vi "Config PM Modulation.vi"(0 "VISA Resource Name":refnum<visa-resource-name>, 1 "Path (0:1)":enum16{"1", "2"}(ring), 2 "Status (T:ON)":bool=TRUE, 3 "EXT Source Coupling (T:AC)":bool=TRUE, 4 "PM Deviation Couple (F:OFF)":bool, 5 "error in (no error)":errorcluster {"code" format="%.0x"}, 6 "PM Deviation (0.0)":dbl format="%.3f", 7 "Dual/Swept Parameters":T1={"Alt Frequency (400.0)"=400.0, "Alt Freq Amplitude (50.0)"=50.0, "Sweep Time (100.0)"=100.0, "Sweep Trigger (0:IMMEDIATE)"=enum."IMMEDIATE"} {"Sweep Time (100.0)" format="%.1f"; "Alt Freq Amplitude (50.0)" format="%.1f"; "Alt Frequency (400.0)" format="%.1f"}, 8 "PM Source (0:Internal)":enum16{"INTERNAL", "EXT1", "EXT2"}(ring), 9 "Bandwidth (T:NORMAL)":bool=TRUE, 10 "PM Rate (400.0)":dbl=400.0 format="%.1f", 12 "PM Waveform (0:SINE)":T2(ring)) -> (14 "VISA Resource Name Out":refnum<visa-resource-name>, 19 "error out":errorcluster {"code" format="%.0x"})   [LabVIEW 2012, in "Agilent ESG Series.lvlib"]
doc: "This VI is used to set the modulation controls and the parameters associated with phase modulated signals."
uses:
  <instrlib>/Agilent ESG Series/Agilent ESG Series.lvlib
panel:
  # "NORMAL"
  # "HIGH"
  # "ON"
  # "OFF"
  # "AC"
  # "DC"
  # "ON"
  # "OFF"
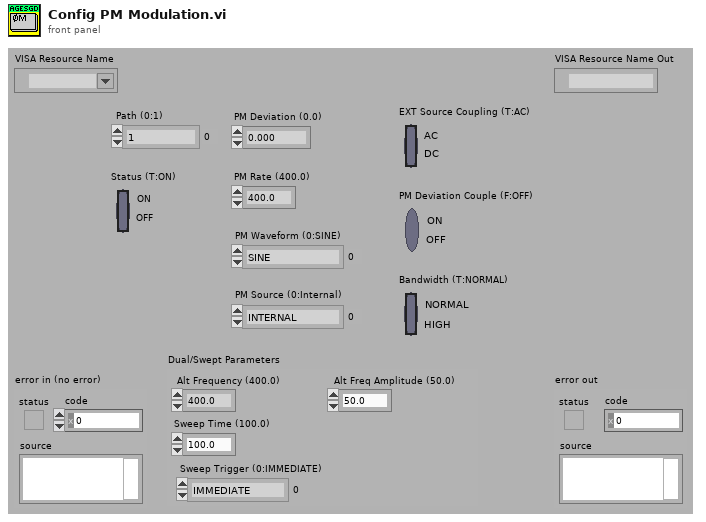
[diagram p1: front panel]
types:
  T1 = cluster{"Alt Frequency (400.0)":dbl, "Alt Freq Amplitude (50.0)":dbl, "Sweep Time (100.0)":dbl, "Sweep Trigger (0:IMMEDIATE)":enum16{"IMMEDIATE", "BUS", "EXTERNAL", "KEY"}}
  T2 = enum16{"SINE", "TRIANGLE", "SQUARE", "RAMP", "NOISE", "DUAL SINE", "SWEPT SINE"}
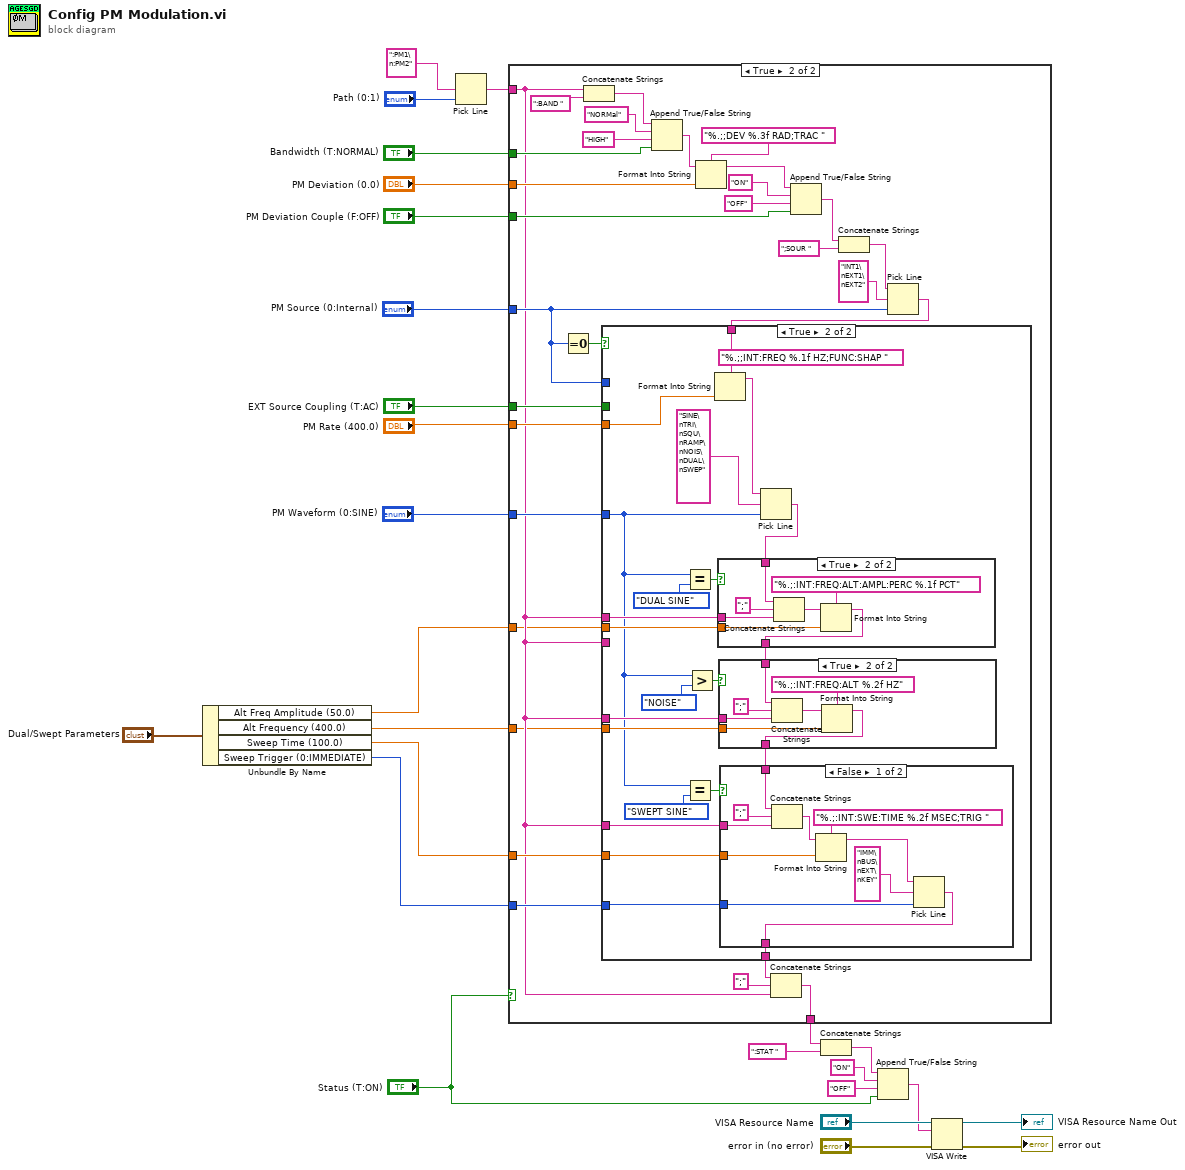
[diagram p0: block diagram]
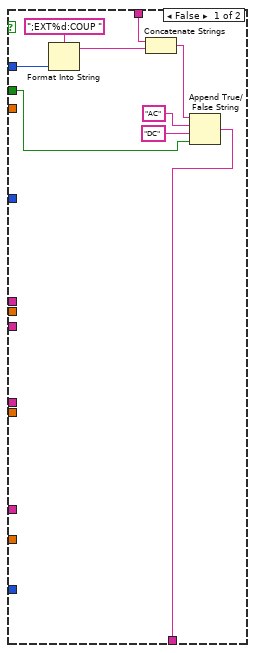
[diagram p3: hidden frame]
diagram:
  n1 = Unbundle By Name("Dual/Swept Parameters") -> ("Alt Freq Amplitude (50.0)"=w3:dbl, "Alt Frequency (400.0)"=w4:dbl, "Sweep Time (100.0)"=w1:dbl, "Sweep Trigger (0:IMMEDIATE)"=w2:enum16{"IMMEDIATE", "BUS", "EXTERNAL", "KEY"})
  n2 = Pick Line(multi-line string=":PM1\n:PM2" ("true string"), line index="Path (0:1)") -> (output string=w9:string)  [unwired: 1 in]
  n3 = case shown="True" "Status (T:ON)" {
    tunnel: "Bandwidth (T:NORMAL)" -> [_ w57]
    tunnel: w9 -> [w27 w30]
    tunnel: [w27 w40] -> w14
    tunnel: w1 -> [_ w38]
    tunnel: w2 -> [_ w37]
    tunnel: "PM Waveform (0:SINE)" -> [_ w36]
    tunnel: "PM Rate (400.0)" -> [_ w35]
    tunnel: "EXT Source Coupling (T:AC)" -> [_ w34]
    tunnel: "PM Source (0:Internal)" -> [_ w33]
    tunnel: "PM Deviation Couple (F:OFF)" -> [_ w32]
    tunnel: "PM Deviation (0.0)" -> [_ w31]
    tunnel: w3 -> [_ w29]
    tunnel: w4 -> [_ w28]
    frame False {
    }
    frame True {
      n4 = Equal To 0?(x=w33) -> (x = 0?=w43:bool)
      n5 = Concatenate Strings(w30, ":BAND ") -> (w55:string)
      n6 = Append True/False String(1:w57, 2:"HIGH" ("false string"), 3:"NORMal" ("true string"), 4:w55) -> (0:w56:string)
      n7 = Format Into String(format string="%.;;DEV %.3f RAD;TRAC ", initial string=w56, w31) -> (resulting string=w48:string)  [unwired: 1 in, 1 out]
      n8 = Append True/False String(1:w32, 2:"OFF" ("false string"), 3:"ON" ("true string"), 4:w48) -> (0:w47:string)
      n9 = Concatenate Strings(w47, ";SOUR ") -> (w45:string)
      n10 = Pick Line(string ("")=w45, multi-line string="INT1\nEXT1\nEXT2", line index=w33) -> (output string=w42:string)
      n11 = case shown="True" w43 {
        tunnel: w42 -> [w65 w89]
        tunnel: [w62 w82] -> w39
        tunnel: w33 -> [w61 _]
        tunnel: w34 -> [w58 _]
        tunnel: w35 -> [_ w88]
        tunnel: w36 -> [_ w69]
        tunnel: w37 -> [_ w80]
        tunnel: w38 -> [_ w81]
        tunnel: w30 -> [_ _]
        tunnel: w30 -> [_ w79]
        tunnel: w30 -> [_ w73]
        tunnel: w30 -> [_ w72]
        tunnel: w29 -> [_ w71]
        tunnel: w28 -> [_ w70]
        frame False {
          n12 = Format Into String(format string=";EXT%d:COUP ", w61) -> (resulting string=w59:string)  [unwired: 2 in, 1 out]
          n13 = Concatenate Strings(w65, w59) -> (w64:string)
          n14 = Append True/False String(1:w58, 2:"DC" ("false string"), 3:"AC" ("true string"), 4:w64) -> (0:w62:string)
        }
        frame True {
          n15 = Equal?(x=w69, y=T2."DUAL SINE") -> (x = y?=w77:bool)
          n16 = Equal?(x=w69, y=T2."SWEPT SINE") -> (x = y?=w83:bool)
          n17 = Greater?(x=w69, y=T2."NOISE") -> (0:w74:bool)
          n18 = Format Into String(format string="%.;;INT:FREQ %.1f HZ;FUNC:SHAP ", initial string=w89, w88) -> (resulting string=w85:string)  [unwired: 1 in, 1 out]
          n19 = Pick Line(string ("")=w85, multi-line string="SINE\nTRI\nSQU\nRAMP\nNOIS\nDUAL\nSWEP", line index=w69) -> (output string=w67:string)
          n20 = case shown="True" w77 {
            tunnel: [w98 w102] -> w75
            tunnel: w67 -> [w98 w101]
            tunnel: w73 -> [_ w100]
            tunnel: w71 -> [_ w99]
            frame False {
            }
            frame True {
              n21 = Concatenate Strings(w101, ";" ("true string"), w100) -> (w104:string)
              n22 = Format Into String(format string="%.;:INT:FREQ:ALT:AMPL:PERC %.1f PCT", initial string=w104, w99) -> (resulting string=w102:string)  [unwired: 1 in, 1 out]
            }
          }
          n23 = case shown="True" w74 {
            tunnel: w75 -> [w90 w94]
            tunnel: [w90 w93] -> w68
            tunnel: w72 -> [_ w92]
            tunnel: w70 -> [_ w91]
            frame False {
            }
            frame True {
              n24 = Concatenate Strings(w94, ";" ("true string"), w92) -> (w96:string)
              n25 = Format Into String(format string="%.;:INT:FREQ:ALT %.2f HZ", initial string=w96, w91) -> (resulting string=w93:string)  [unwired: 1 in, 1 out]
            }
          }
          n26 = case shown="False" w83 {
            tunnel: w68 -> [w106 w116]
            tunnel: [w112 w116] -> w82
            tunnel: w81 -> [w111 _]
            tunnel: w80 -> [w110 _]
            tunnel: w79 -> [w108 _]
            frame False {
              n27 = Concatenate Strings(w106, ";" ("true string"), w108) -> (w107:string)
              n28 = Format Into String(format string="%.;:INT:SWE:TIME %.2f MSEC;TRIG ", initial string=w107, w111) -> (resulting string=w115:string)  [unwired: 1 in, 1 out]
              n29 = Pick Line(string ("")=w115, multi-line string="IMM\nBUS\nEXT\nKEY", line index=w110) -> (output string=w112:string)
            }
            frame True {
            }
          }
        }
      }
      n30 = Concatenate Strings(w39, ";" ("true string"), w30) -> (w40:string)
    }
  }
  n31 = Concatenate Strings(w14, ":STAT ") -> (w12:string)
  n32 = Append True/False String(1:"Status (T:ON)", 2:"OFF" ("false string"), 3:"ON" ("true string"), 4:w12) -> (0:w6:string)
  n33 = VISA Write(VISA resource name="VISA Resource Name", write buffer=w6, error in (no error)="error in (no error)") -> (VISA resource name out=→"VISA Resource Name Out":refnum<visa-resource-name>, error out=→"error out":errorcluster)  [unwired: 1 out]
